vi "Probe.vi"(8 "error in (no error)":errorcluster, 10 "Buffer":u8[](array[numeric]), 11 "LEN in":refnum<class "LEN.lvclass">) -> (0 "error out":errorcluster, 1 "Valid":bool, 2 "Buffer Count":i32, 3 "LEN out":refnum<class "LEN.lvclass">)   [LabVIEW 2020, in "Protobuf RAW.lvlib" / "LEN.lvclass"]
uses:
  LEN.lvclass
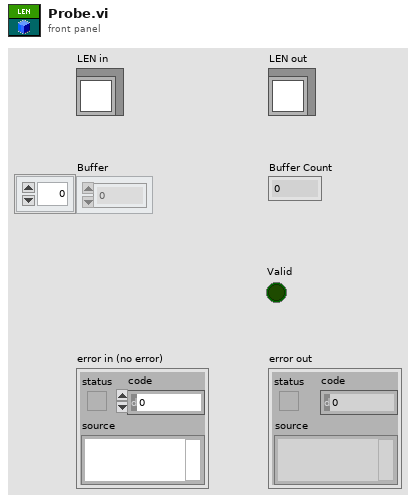
[diagram p1: front panel]
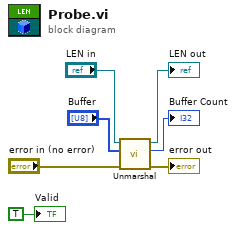
[diagram p0: block diagram]
diagram:
  n1 = call-dynamic "Unmarshal.vi"("error in (no error)"="error in (no error)", "Buffer"="Buffer", "LEN in"="LEN in") -> ("error out"=→"error out":errorcluster, "Buffer Count"=→"Buffer Count":i32, "LEN out"=→"LEN out":refnum<class "LEN.lvclass">)  [unwired: 6 in]
  "Valid" <- TRUE ("Valid")
